vi "Autosampler Prime Pump.vi"(6 "Cycles":u16=5, 7 "Correlation ID":u32, 8 "error in (no error)":errorcluster, 9 "Waste Valve Pos.":u16=2, 10 "Buffer Val Pos.":u16=3, 11 "Application in":refnum<class "Application.lvclass">) -> (0 "error out":errorcluster, 3 "Application out":refnum<class "Application.lvclass">)   [LabVIEW 2023, in "Application.lvlib" / "Application.lvclass"]
uses:
  Application.lvclass
  Application.lvclass/Application.ctl
  Hardware/Device Messages/Save CorrID Msg/Save CorrID Msg.lvclass/Save CorrID Msg.ctl
  <vilib>/ActorFramework/Message Enqueuer/Message Enqueuer.lvclass/Message Enqueuer.ctl
  Hardware/Autosampler Messages/Prime Pump Msg/Prime Pump Msg.lvclass/Prime Pump Msg.ctl
  <vilib>/ActorFramework/Message Enqueuer/Enqueue.vi
  Hardware/Device Messages/Save CorrID Msg/Save CorrID Msg.lvclass
  Hardware/Autosampler Messages/Prime Pump Msg/Prime Pump Msg.lvclass
  <vilib>/ActorFramework/Message Priority Queue/Priority Enqueue.vi
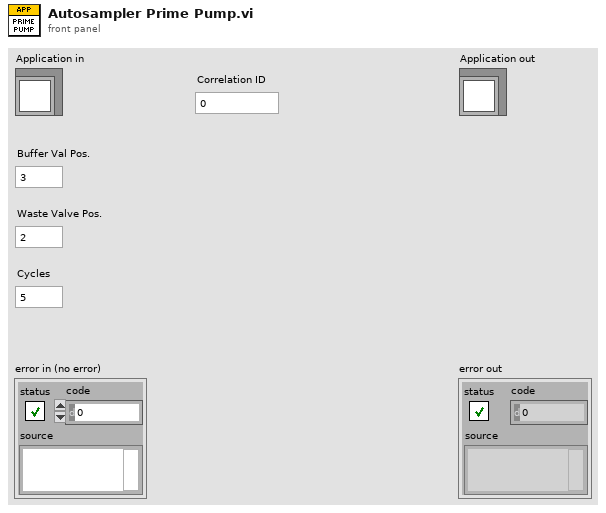
[diagram p1: front panel]
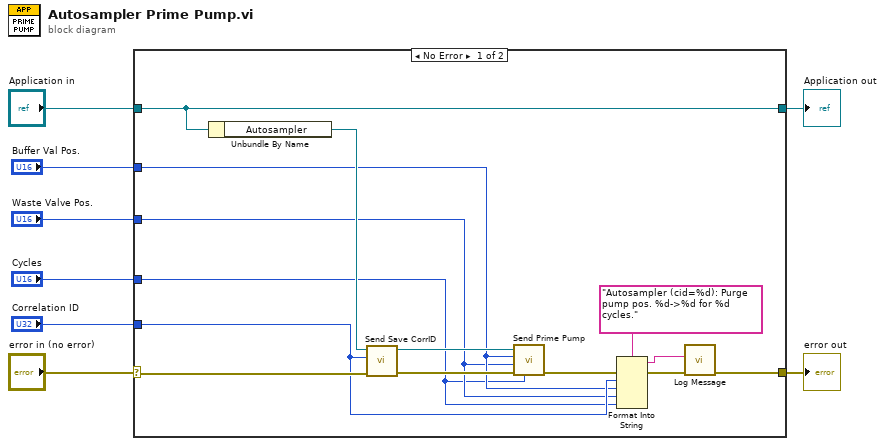
[diagram p0: block diagram]
diagram:
  n1 = case shown="No Error" "error in (no error)" {
    selector: "error in (no error)" -> [w18 w24]
    tunnel: [w13 w24] -> w7
    tunnel: [w22 w23] -> w5
    tunnel: "Application in" -> [w22 w23]
    tunnel: "Cycles" -> [w9 _]
    tunnel: "Waste Valve Pos." -> [w10 _]
    tunnel: "Buffer Val Pos." -> [w11 _]
    tunnel: "Correlation ID" -> [w12 _]
    frame No Error {
      n2 = Unbundle By Name(w22) -> ("Autosampler"=w16:refnum<class "Message Enqueuer.lvclass">)
      n3 = call "Send Save CorrID.vi"("error in (no error)"=w18, "Correlation ID"=w12, "Message Enqueuer"=w16) -> ("error out"=w17:errorcluster, "Message Enqueuer out"=w15:refnum<class "Message Enqueuer.lvclass">)  [unwired: 7 in]
      n4 = call "Send Prime Pump.vi"("Cycles"=w9, "error in (no error)"=w17, "Waste Valve Pos."=w10, "Buffer Val Pos."=w11, "Message Enqueuer"=w15) -> ("error out"=w14:errorcluster)  [unwired: 5 in, 1 out]
      n5 = Format Into String(format string="Autosampler (cid=%d): Purge pump pos. %d->%d for %d cycles.", error in=w14, w12, w11, w10, w9) -> (resulting string=w21:string, error out=w20:errorcluster)  [unwired: 1 in]
      n6 = call "Log Message.vi"("error constant"=w20, "input"=w21) -> ("error constant 2"=w13:errorcluster)  [unwired: 8 in, 1 out]
    }
    frame Error {
    }
  }
  "error out" <- w7
  "Application out" <- w5
